vi "計時器+閃爍.vi"(4 "時間設定":dbl format="%#.6f", 6 "動作":bool) -> (0 "時間到":bool, 1 "°{Ã{":bool, 2 "計數時間":dbl format="%.2f", 3 "開始時間":dbl format="%.2f")   [LabVIEW 2015]
panel:
  in  "Hold":bool
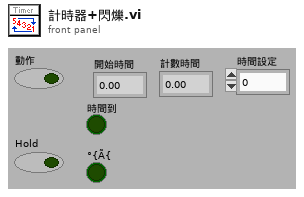
[diagram p1: front panel]
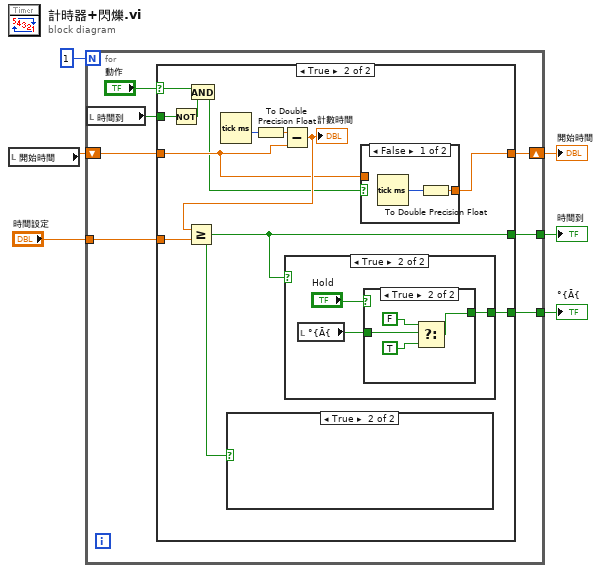
[diagram p0: block diagram]
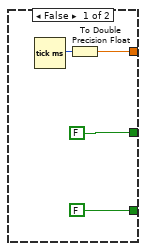
[diagram p2: hidden frame]
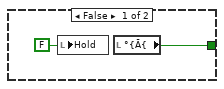
[diagram p4: hidden frame]
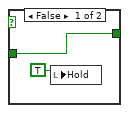
[diagram p5: hidden frame]
diagram:
  n1 = local read "開始時間"() -> (w4:dbl)
  n2 = for {
    N: 1 -> [_]
    shift-right: [w12] -> w5
    shift-left: w4 -> [w13]
    tunnel: "時間設定" -> [w10]
    tunnel: [w7] -> w1
    tunnel: [w9] -> w2
    n3 = local read "時間到"() -> (w8:bool)
    n4 = case shown="True" "動作" {
      selector: "動作" -> [_ w24]
      tunnel: w13 -> [_ w26]
      tunnel: [w17 w27] -> w12
      tunnel: w10 -> [_ w25]
      tunnel: [FALSE w18] -> w9
      tunnel: w8 -> [_ w23]
      tunnel: [FALSE ("°{Ã{") w20] -> w7
      frame False {
        n5 = Tick Count (ms)() -> (millisecond timer value=w14:u32)
        n6 = To Double Precision Float(number=w14) -> (double precision float=w17:dbl)
      }
      frame True {
        n7 = Not(x=w23) -> (.not. x?=w22:bool)
        n8 = And(x=w24, y=w22) -> (x .and. y?=w21:bool)
        n9 = Tick Count (ms)() -> (millisecond timer value=w19:u32)
        n10 = To Double Precision Float(number=w19) -> (double precision float=w29:dbl)
        n11 = Subtract(x=w29, y=w26) -> (x-y=w28:dbl)
        "計數時間" <- w28
        n12 = Greater Or Equal?(x=w28, y=w25) -> (x >= y?=w18:bool)
        n13 = case shown="True" w18 {
          frame False {
          }
          frame True {
          }
        }
        n14 = case shown="True" w18 {
          tunnel: [w30 w34] -> w20
          frame False {
            n15 = local write "Hold"(FALSE ("Hold")) -> ()
            n16 = local read "°{Ã{"() -> (w30:bool)
          }
          frame True {
            n17 = local read "°{Ã{"() -> (w33:bool)
            n18 = case shown="True" "Hold" {
              tunnel: [w35 w38] -> w34
              tunnel: w33 -> [w35 w40]
              frame False {
                n19 = local write "Hold"(TRUE ("Hold")) -> ()
              }
              frame True {
                n20 = Select(t=FALSE ("°{Ã{"), s=w40, f=TRUE ("°{Ã{")) -> (s? t:f=w38:bool)
              }
            }
          }
        }
        n21 = case shown="False" w21 {
          tunnel: [w42 w43] -> w27
          tunnel: w26 -> [_ w43]
          frame False {
            n22 = Tick Count (ms)() -> (millisecond timer value=w41:u32)
            n23 = To Double Precision Float(number=w41) -> (double precision float=w42:dbl)
          }
          frame True {
          }
        }
      }
    }
  }
  "開始時間" <- w5
  "時間到" <- w2
  "°{Ã{" <- w1
